vi "create safe outputs command.vi"(9 "Safe Voltage":fxp<+/-,20,5>[](array[numeric])=[0.0, 0.0, 0.0, 0.0], 11 "Safe Digital":bool[](array[boolean])=[FALSE, FALSE, FALSE, FALSE, FALSE, FALSE, FALSE, FALSE]) -> (3 "command message":variant)   [LabVIEW 2018]
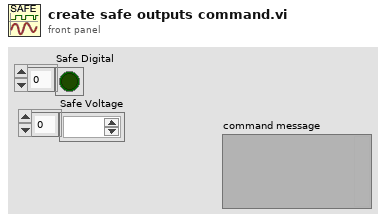
[diagram p1: front panel]
types:
  T1 = cluster{"Safe Digital":bool[], "Safe Voltage":fxp<+/-,20,5>[]}
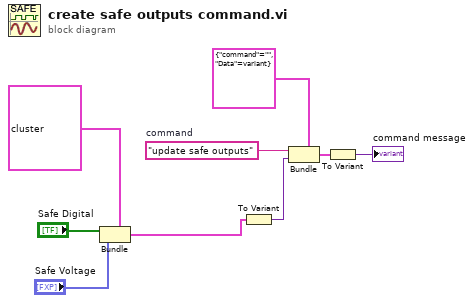
[diagram p0: block diagram]
diagram:
  w8 = "update safe outputs"  # command
  n1 = Bundle(cluster=T1 {"Safe Digital"=[FALSE, FALSE, FALSE, FALSE, FALSE, FALSE, FALSE, FALSE], "Safe Voltage"=[0.0, 0.0, 0.0, 0.0]}, "Safe Digital"="Safe Digital", "Safe Voltage"="Safe Voltage") -> (w3:T1)
  n2 = To Variant(anything=w3) -> (Variant=w7:variant)
  n3 = Bundle(cluster=cluster{"command":string, "Data":variant} {"command"="", "Data"=variant}, "command"=w8, "Data"=w7) -> (w6:cluster{"command":string, "Data":variant})
  n4 = To Variant(anything=w6) -> (Variant=→"command message":variant)
